vi "Initialize.vi"(8 "error in (no error)":errorcluster, 11 "SecMirror in":refnum<class "SecMirror.lvclass">) -> (0 "error out":errorcluster, 3 "SecMirror out":refnum<class "SecMirror.lvclass">)   [LabVIEW 2018, in "SecMirror.lvclass"]
uses:
  SecMirror.lvclass
  Device/Device.lvclass
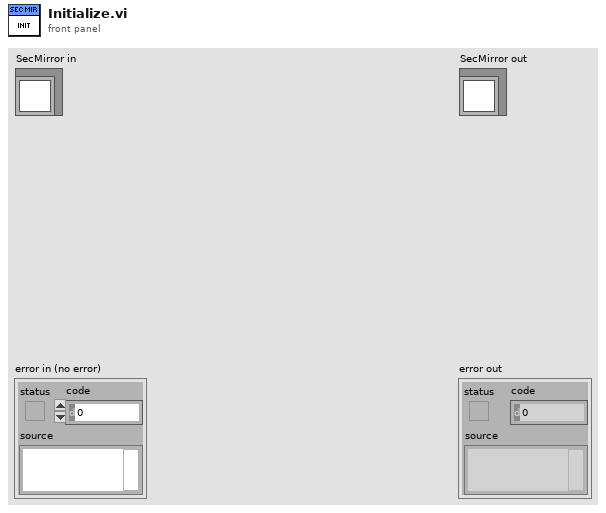
[diagram p1: front panel]
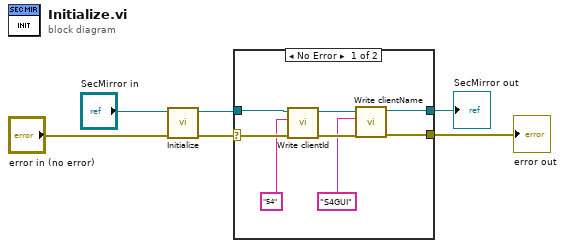
[diagram p0: block diagram]
diagram:
  n1 = call-parent "Initialize.vi"("error in (no error)"="error in (no error)", "Device in"="SecMirror in") -> ("error out"=w4:errorcluster, "Device out"=w3:refnum<class "SecMirror.lvclass">)  [unwired: 8 in]
  n2 = case shown="No Error" w4 {
    selector: w4 -> [w14 w15]
    tunnel: [w9 w16] -> w2
    tunnel: w3 -> [w11 w16]
    tunnel: [w12 w15] -> w1
    frame No Error {
      n3 = call-dynamic "Write clientId.vi"("error in (no error)"=w14, "clientId"="54", "Device in"=w11) -> ("error out"=w13:errorcluster, "Device out"=w10:refnum<class "SecMirror.lvclass">)  [unwired: 7 in]
      n4 = call-dynamic "Write clientName.vi"("error in (no error)"=w13, "clientName"="S4GUI", "Device in"=w10) -> ("error out"=w12:errorcluster, "Device out"=w9:refnum<class "SecMirror.lvclass">)  [unwired: 7 in]
    }
    frame Error {
    }
  }
  "error out" <- w1
  "SecMirror out" <- w2
